vi "resetSettledCheck.vi"(8 "error in (no error)":errorcluster, 10 "loopPeriod":dbl[unit]=5000.0 min=10.0 max=5000.0, 11 "SystemController in":refnum<class "SystemController.lvclass">) -> (0 "error out":errorcluster, 2 "settledIsTrue":bool, 3 "SystemController out":refnum<class "SystemController.lvclass">)   [LabVIEW 2015, in "SystemController.lvclass"]
uses:
  SystemController.lvclass
  SystemController.lvclass/SystemController.ctl
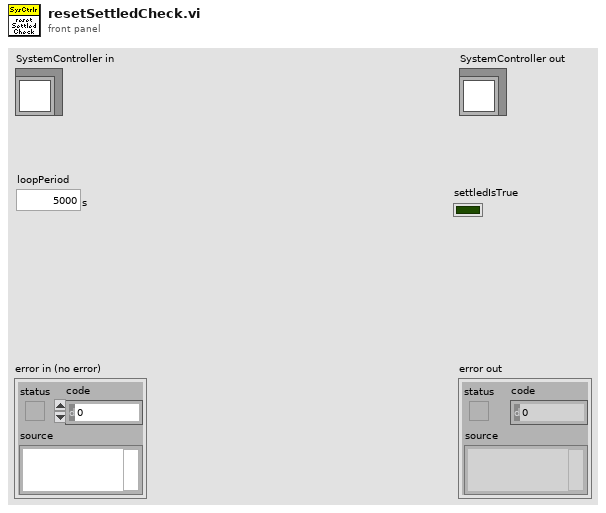
[diagram p1: front panel]
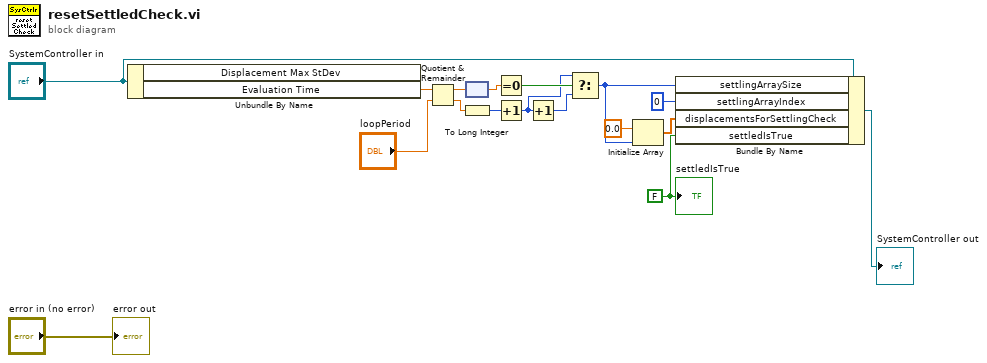
[diagram p0: block diagram]
diagram:
  w1 = FALSE ("settledIsTrue")
  n1 = Unbundle By Name("SystemController in") -> ("Evaluation Time"=w12:dbl[unit])  [unwired: 1 out]
  n2 = Quotient & Remainder(x=w12, y="loopPeriod") -> (x-y*floor(x/y)=w10:dbl[unit], floor(x/y)=w5:dbl)
  n3 = To Long Integer(number=w5) -> (32bit integer=w4:i32)
  n4 = node(w10) -> (w9:dbl)
  n5 = Equal To 0?(x=w9) -> (x = 0?=w8:bool)
  n6 = Increment(x=w4) -> (x+1=w6:i32)
  n7 = Increment(x=w6) -> (x+1=w7:i32)
  n8 = Select(t=w6, s=w8, f=w7) -> (s? t:f=w2:i32)
  n9 = Initialize Array(dbl[unit] 0.0 ("element"), w2) -> (w3:dbl[unit][])
  n10 = Bundle By Name(cluster="SystemController in", "settlingArraySize"=w2, "settlingArrayIndex"=0, "displacementsForSettlingCheck"=w3, "settledIsTrue"=w1) -> (→"SystemController out":refnum<class "SystemController.lvclass">)
  "error out" <- "error in (no error)"
  "settledIsTrue" <- w1
